vi "Test akwizycji 2.vi"() -> ()   [LabVIEW 2014]
uses:
  Kontrolki/KartaDAQ/ACQ all read tasks.ctl
  Kontrolki/KartaDAQ/ACQ analog channel config new.ctl
  Kontrolki/KartaDAQ/ACQ Params.ctl
  Kontrolki/KartaDAQ/ACQ counter channel config.ctl
panel:
  out "Waveform Graph":waveform(dbl)[](graph)
  in  "stop":bool
  in  "Urz¹dzenie":tag="Dev1"
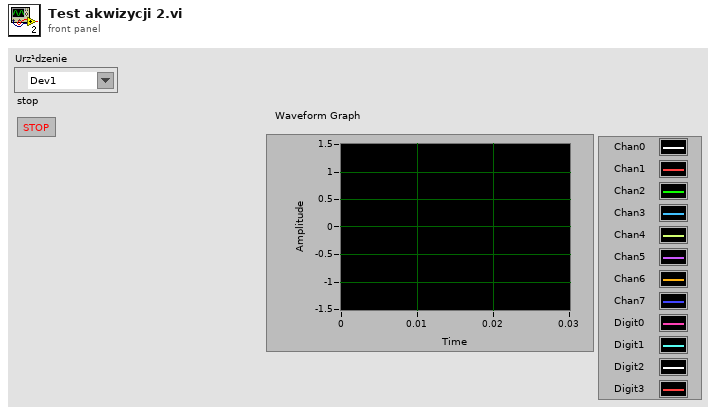
[diagram p1: front panel]
types:
  T1 = typedef "ACQ counter channel config.ctl" = cluster{"Enkoder X":string, "Enkoder Y":string, "Generator":string, "Generator OUT":string}
  T2 = typedef "ACQ Params.ctl" = cluster{"Analog":cluster{"minimum value":dbl, "maximum value":dbl}, "Digital":cluster{"minimum value":dbl, "maximum value":dbl}, "Time":cluster{"sample mode":i32, "samples per channel in":i32, "rate":dbl, "active edge":i32}, "AI common":cluster{"input terminal configuration":i32, "source":string}, "Enkoder":cluster{"channel1 name":string, "channel2 name":string, "units":i32, "initial position":dbl, "distance per pulse":dbl, "z index enable":bool, "z index value":dbl, "z index phase":i32, "decoding type":i32}}
  T3 = typedef "ACQ analog channel config new.ctl" = cluster{"Analogs IN":string[], "Digitals IN":string[]}
  T4 = typedef "ACQ all read tasks.ctl" = cluster{"Analog ref":refnum<k21>, "Enkoder X ref":refnum<k21>, "Enkoder Y ref":refnum<k21>, "Generator ref":refnum<k21>}
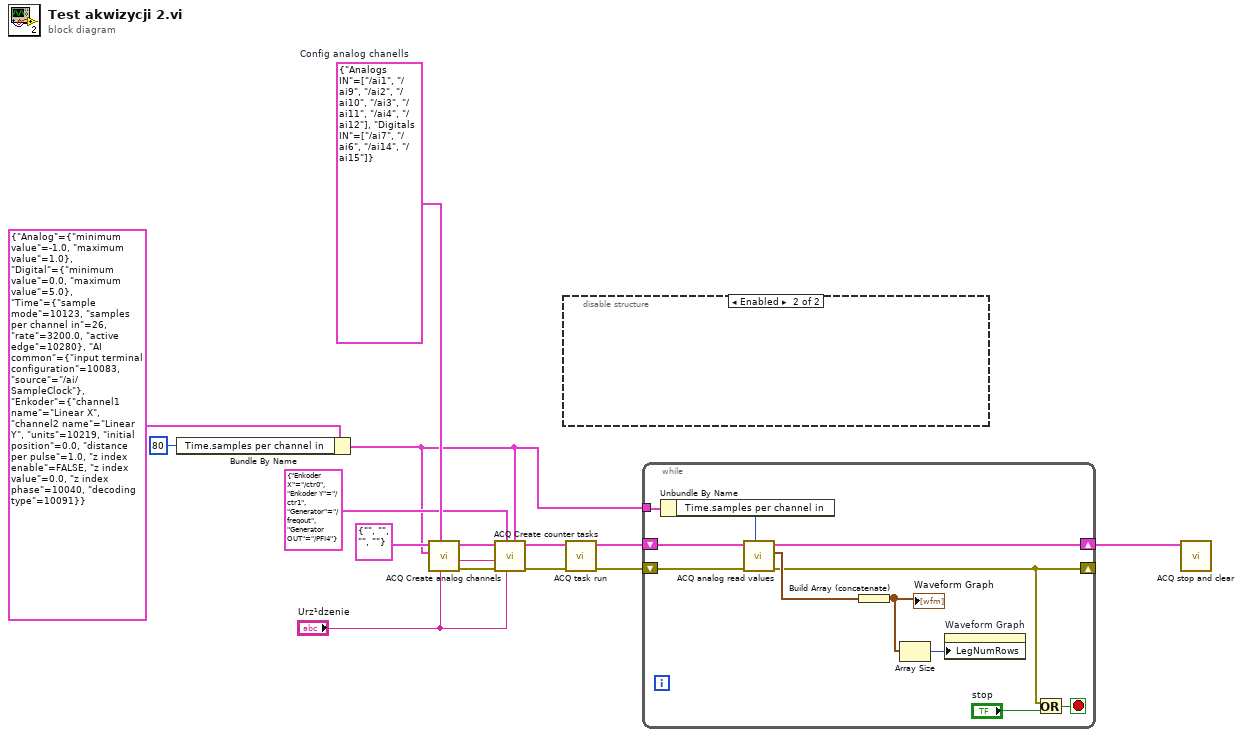
[diagram p0: block diagram]
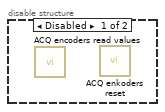
[diagram p2: hidden frame]
diagram:
  w14 = T3 {"Analogs IN"=["/ai1", "/ai9", "/ai2", "/ai10", "/ai3", "/ai11", "/ai4", "/ai12"], "Digitals IN"=["/ai7", "/ai6", "/ai14", "/ai15"]}  # Config analog chanells
  n1 = Bundle By Name(cluster=T2 {"Analog"={"minimum value"=-1.0, "maximum value"=1.0}, "Digital"={"minimum value"=0.0, "maximum value"=5.0}, "Time"={"sample mode"=10123, "samples per channel in"=26, "rate"=3200.0, "active edge"=10280}, "AI common"={"input terminal configuration"=10083, "source"="/ai/SampleClock"}, "Enkoder"={"channel1 name"="Linear X", "channel2 name"="Linear Y", "units"=10219, "initial position"=0.0, "distance per pulse"=1.0, "z index enable"=FALSE, "z index value"=0.0, "z index phase"=10040, "decoding type"=10091}} ("ACQ Params"), "Time.samples per channel in"=80) -> (w2:T2)
  n2 = call "ACQ Create analog channels.vi"("device in"="Urz¹dzenie", "Config analog chanells new"=w14, "ACQ Params"=w2, "All Read tasks in"=T4 {"Analog ref"="", "Enkoder X ref"="", "Enkoder Y ref"="", "Generator ref"=""}) -> ("error out"=w11:errorcluster, "Terminal Name with Device Prefix"=w10:tag, "All Read tasks out"=w12:T4)  [unwired: 4 in, 1 out]
  n3 = call "ACQ Create counter tasks.vi"("ACQ Params"=w2, "device in"="Urz¹dzenie", "Config Counter channels"=T1 {"Enkoder X"="/ctr0", "Enkoder Y"="/ctr1", "Generator"="/freqout", "Generator OUT"="/PFI4"}, "error in (no error)"=w11, "Terminal Name with Device Prefix"=w10, "All Read tasks in"=w12) -> ("error out"=w9:errorcluster, "All Read tasks out"=w8:T4)  [unwired: 4 in]
  n4 = disable-structure shown="Enabled" {
    frame Disabled {
      n5 = call "ACQ encoders read values.vi"() -> ()  [unwired: 9 in, 3 out]
      n6 = call "ACQ enkoders reset.vi"() -> ()  [unwired: 10 in, 2 out]
    }
    frame Enabled {
    }
  }
  n7 = call "ACQ task run.vi"("error in (no error)"=w9, "All Read tasks in"=w8) -> ("error out"=w7:errorcluster, "All Read tasks out"=w6:T4)  [unwired: 7 in, 1 out]
  n8 = while {
    shift-right: [w17] -> w15
    shift-left: w6 -> [w21]
    shift-right: [w16] -> _
    shift-left: w7 -> [w22]
    tunnel: w2 -> [w23]
    stop <- w25 stop-if-true
    n9 = Unbundle By Name(w23) -> ("Time.samples per channel in"=w20:i32)
    n10 = call "ACQ analog read values.vi"("samples per channel"=w20, "error in (no error)"=w22, "Tasks ref in"=w21) -> ("error out"=w16:errorcluster, "data"=w19:waveform(dbl)[], "Tasks ref out"=w17:T4)  [unwired: 6 in]
    n11 = Build Array (concatenate)(w19) -> (w18:waveform(dbl)[])
    "Waveform Graph" <- w18
    n12 = Array Size(array=w18) -> (size(s)=w26:i32)
    n13 = property on="Waveform Graph" class="WFGraph (strict)"("LegNumRows"=w26) -> ()  [unwired: 2 in, 2 out]
    n14 = Or(x=w16, y="stop") -> (x .or. y?=w25:bool)
  }
  n15 = call "ACQ stop and clear.vi"("Tasks ref in"=w15) -> ()  [unwired: 10 in, 1 out]
